vi "RPC Method PerformOCVMeasurement.vi"(8 "error in (no error)":errorcluster, 11 "OOP Server in":refnum<class "OCV2.lvclass">) -> (0 "error out":errorcluster, 3 "OOP Server out":refnum<class "OCV2.lvclass">)   [LabVIEW 2019, in "OCV2.lvlib" / "OCV2.lvclass"]
uses:
  OCV2.lvclass
  OCV2.lvclass/OCV2.ctl
  RPC Messages/measurementservice_ErrorOut/measurementservice_ErrorOut_Data.ctl
  RPC Messages/measurementservice_OCVRaw/measurementservice_OCVRaw_Data.ctl
  RPC Messages/measurementservice_OCVData/measurementservice_OCVData_Data.ctl
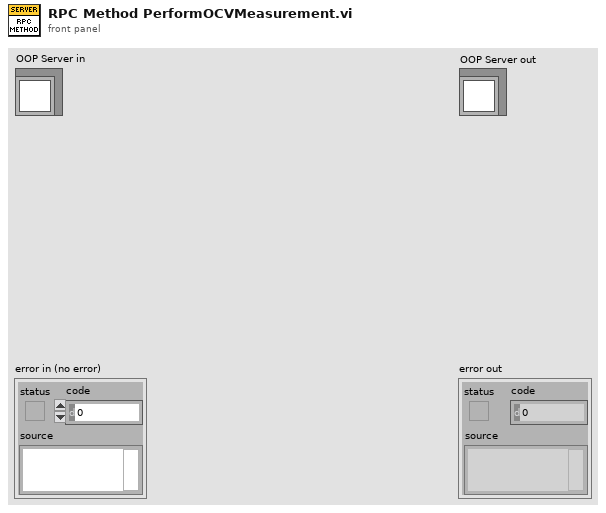
[diagram p1: front panel]
types:
  T1 = typedef "OCV2.lvlib/OCV2.lvclass/measurementservice_OCVData_Data.ctl" = cluster{"data":T2[]}
  T2 = typedef "OCV2.lvlib/OCV2.lvclass/measurementservice_OCVRaw_Data.ctl" = cluster{"battery1voltage":sgl, "battery2voltage":sgl, "battery3voltage":sgl, "battery4voltage":sgl, "battery5voltage":sgl, "battery6voltage":sgl, "battery7voltage":sgl, "battery8voltage":sgl, "battery9voltage":sgl, "battery10voltage":sgl, "battery11voltage":sgl, "battery12voltage":sgl, "battery13voltage":sgl, "battery14voltage":sgl, "battery15voltage":sgl, "battery16voltage":sgl, "battery17voltage":sgl, "battery18voltage":sgl, "battery19voltage":sgl, "battery20voltage":sgl, "battery21voltage":sgl, "battery22voltage":sgl, "battery23voltage":sgl, "battery24voltage":sgl, "error":T3}
  T3 = typedef "OCV2.lvlib/OCV2.lvclass/measurementservice_ErrorOut_Data.ctl" = cluster{"errCode":i32, "errMessage":string}
  T4 = typedef "OCV2.lvlib/OCV2.lvclass/Server Internal UEs.ctl" = cluster{"Invoke Internal UE":refnum<user-event>, "Query Internal UE":refnum<user-event>, "PerformOCVMeasurement Internal UE":refnum<user-event>, "PerformACIRMeasurement Internal UE":refnum<user-event>, "StreamOCVMeasurement Internal UE":refnum<user-event>, "Register Internal UE":refnum<user-event>}
  T5 = typedef "OCV2.lvlib/OCV2.lvclass/Server gRPC UEs.ctl" = cluster{"Invoke gRPC UE":refnum<user-event>, "Query gRPC UE":refnum<user-event>, "PerformOCVMeasurement gRPC UE":refnum<user-event>, "PerformACIRMeasurement gRPC UE":refnum<user-event>, "StreamOCVMeasurement gRPC UE":refnum<user-event>, "Register gRPC UE":refnum<user-event>}
  T6 = typedef "OCV2.lvlib/gprc-lvsupport.lvlib/grpcId.ctl" = u64
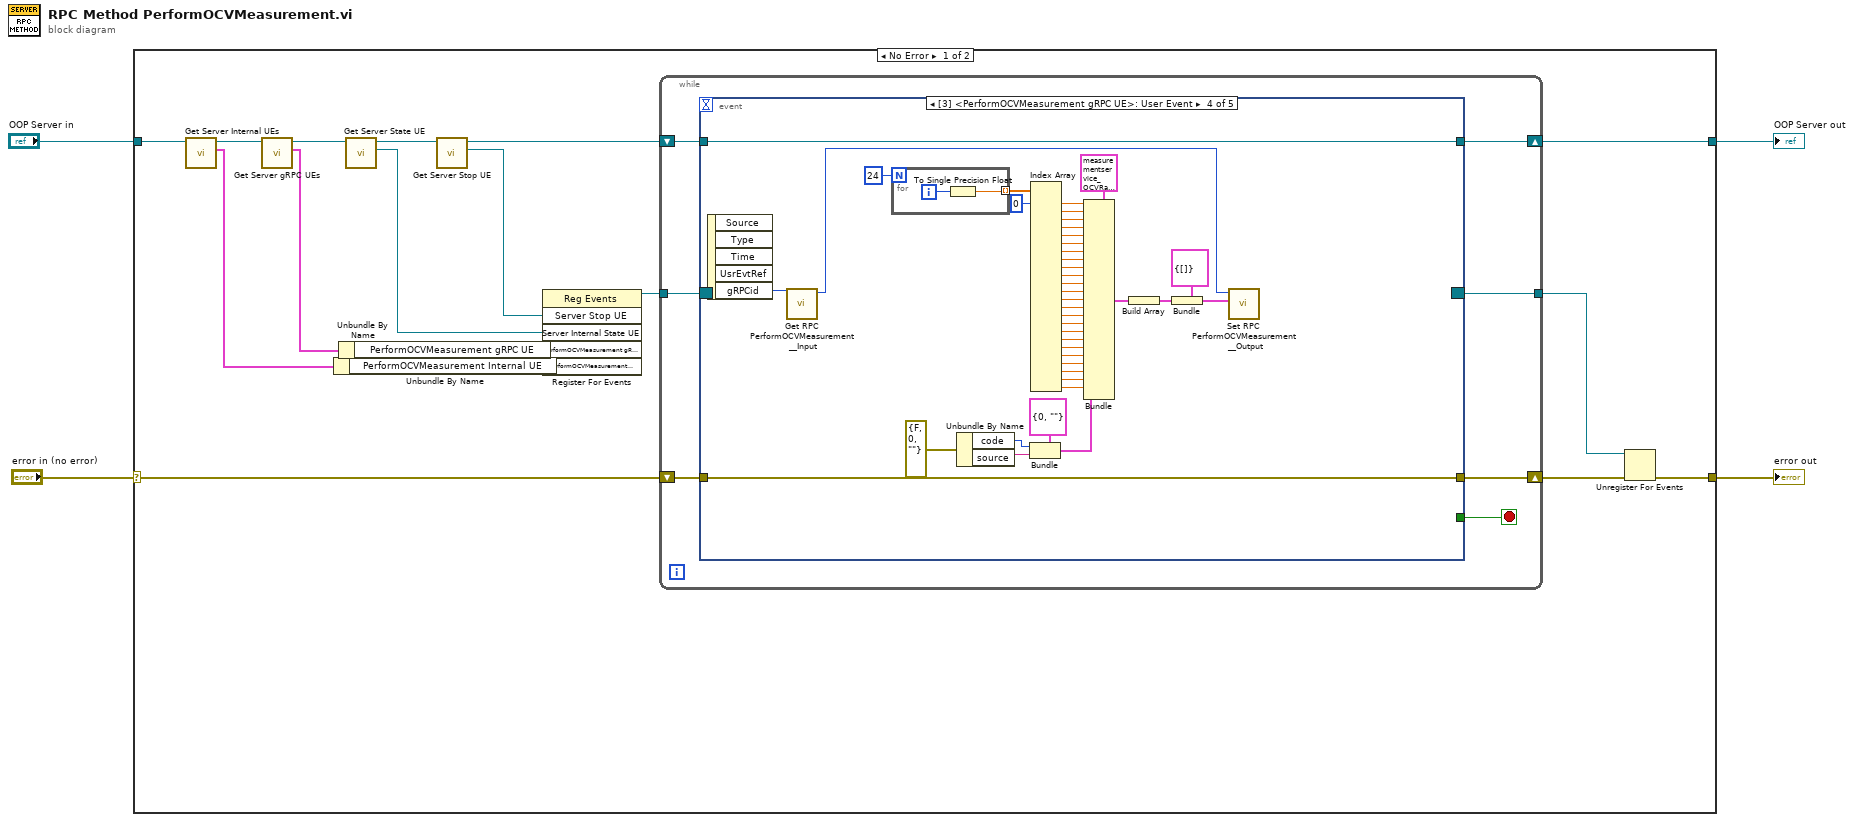
[diagram p0: block diagram]
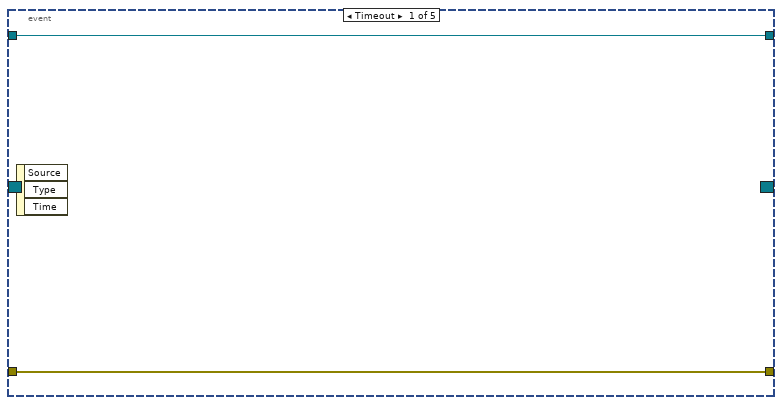
[diagram p2: hidden frame]
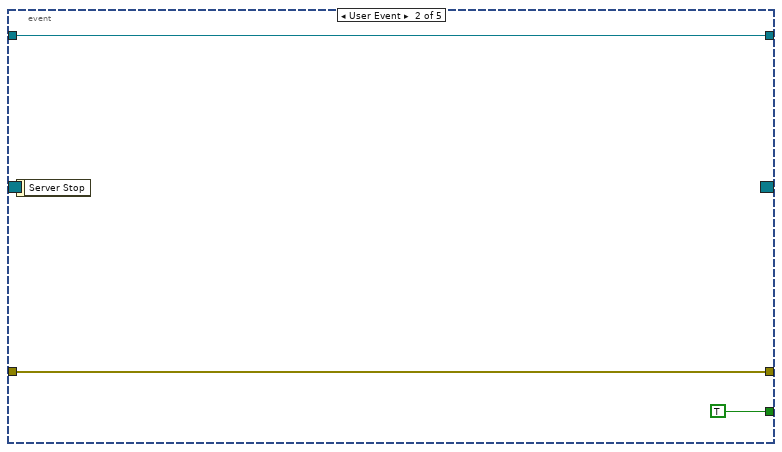
[diagram p3: hidden frame]
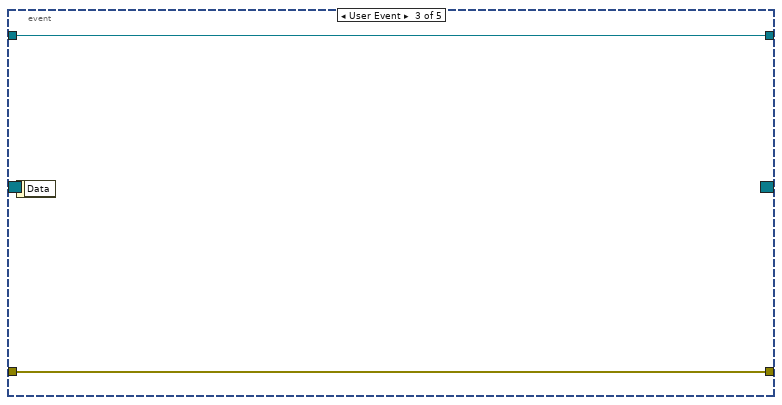
[diagram p4: hidden frame]
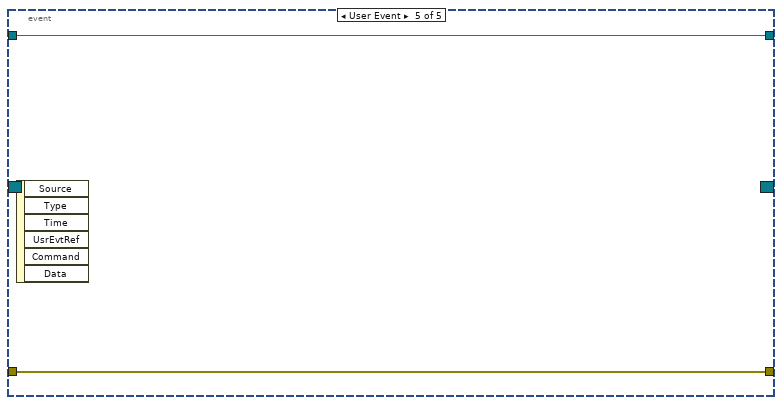
[diagram p5: hidden frame]
diagram:
  n1 = case shown="No Error" "error in (no error)" {
    selector: "error in (no error)" -> [w17 w82]
    tunnel: [w15 w82] -> w3
    tunnel: "OOP Server in" -> [w19 w81]
    tunnel: [w5 w81] -> w1
    frame No Error {
      n2 = call "Get Server Internal UEs.vi"("OOP Server in"=w19) -> ("Server Internal UEs"=w11:T4, "OOP Server out"=w18:refnum<class "OCV2.lvclass">)  [unwired: 9 in]
      n3 = call "Get Server gRPC UEs.vi"("OOP Server in"=w18) -> ("Server gRPC UEs"=w13:T5, "OOP Server out"=w8:refnum<class "OCV2.lvclass">)  [unwired: 9 in]
      n4 = Unbundle By Name ("Unbundle Internal UE")(w11) -> ("PerformOCVMeasurement Internal UE"=w10:refnum<user-event>)
      n5 = Unbundle By Name ("Unbundle gRPC UE")(w13) -> ("PerformOCVMeasurement gRPC UE"=w12:refnum<user-event>)
      n6 = call "Get Server State UE.vi"("Template Server in"=w8) -> ("Server Internal State UE"=w6:refnum<user-event>, "Template Server out"=w7:refnum<class "OCV2.lvclass">)  [unwired: 9 in]
      n7 = call "Get Server Stop UE.vi"("OOP Server in"=w7) -> ("Server Stop UE"=w21:refnum<user-event>, "OOP Server out"=w9:refnum<class "OCV2.lvclass">)  [unwired: 9 in]
      n8 = register-events(w21, w6, w12, w10) -> (reference out=w20:refnum<event-registration>)  [unwired: 2 in, 1 out]
      n9 = while {
        tunnel: w20 -> [w28]
        tunnel: [w24] -> w14
        shift-right: [w25] -> w16
        shift-left: w17 -> [w26]
        shift-right: [w22] -> w5
        shift-left: w9 -> [w23]
        stop <- w27 stop-if-true
        n10 = event "RPC Method Event Structure" shown="[3] <PerformOCVMeasurement gRPC UE>: User Event" {
          selector: w28 -> [_ _ _ _ _]
          dyn-events: [_ _ _ _ _] -> w24
          timeout: _ -> [_ _ _ _ _]
          tunnel: [_ TRUE _ _ _] -> w27
          tunnel: w26 -> [w30 w32 w35 w76 w80]
          tunnel: [w30 w32 w35 w76 w80] -> w25
          tunnel: w23 -> [w29 w31 w34 w75 w79]
          tunnel: [w29 w31 w34 w75 w79] -> w22
          event Timeout {
            n11 = event-data() -> ()  [unwired: 1 in, 3 out]
          }
          event User Event {
            n12 = event-data() -> ()  [unwired: 1 in, 1 out]
          }
          event User Event {
            n13 = event-data() -> ()  [unwired: 1 in, 1 out]
          }
          event User Event {
            n14 = event-data() -> ("gRPCid"=w42:T6)  [unwired: 1 in, 4 out]
            n15 = call "Get RPC PerformOCVMeasurement __Input.vi"("gRPCid in"=w42) -> ("gRPCid out"=w41:T6)  [unwired: 8 in, 2 out]
            n16 = for {
              N: 24 -> [_]
              tunnel: [w78] -> w45 mode=indexing
              i -> [w77]
              n17 = To Single Precision Float(number=w77) -> (single precision float=w78:sgl)
            }
            n18 = Unbundle By Name(errorcluster {"status"=FALSE, "code"=0, "source"=""} ("input cluster")) -> ("code"=w72:i32, "source"=w71:string)
            n19 = Bundle(cluster=T3 {"errCode"=0, "errMessage"=""} ("measurementservice_ErrorOut_Data"), "errCode"=w72, "errMessage"=w71) -> (w70:T3)
            n20 = Index Array(array=w45, index #1=0 ("index")) -> (element #1=w69:sgl, element #2=w68:sgl, element #3=w67:sgl, element #4=w66:sgl, element #5=w65:sgl, element #6=w64:sgl, element #7=w63:sgl, element #8=w62:sgl, element #9=w61:sgl, element #10=w60:sgl, element #11=w59:sgl, element #12=w58:sgl, element #13=w57:sgl, element #14=w56:sgl, element #15=w55:sgl, element #16=w54:sgl, element #17=w53:sgl, element #18=w52:sgl, element #19=w51:sgl, element #20=w50:sgl, element #21=w49:sgl, element #22=w48:sgl, element #23=w47:sgl, element #24=w46:sgl)  [unwired: 23 in]
            n21 = Bundle(cluster=T2 {"battery1voltage"=0.0, "battery2voltage"=0.0, "battery3voltage"=0.0, "battery4voltage"=0.0, "battery5voltage"=0.0, "battery6voltage"=0.0, "battery7voltage"=0.0, "battery8voltage"=0.0, "battery9voltage"=0.0, "battery10voltage"=0.0, "battery11voltage"=0.0, "battery12voltage"=0.0, "battery13voltage"=0.0, "battery14voltage"=0.0, "battery15voltage"=0.0, "battery16voltage"=0.0, "battery17voltage"=0.0, "battery18voltage"=0.0, "battery19voltage"=0.0, "battery20voltage"=0.0, "battery21voltage"=0.0, "battery22voltage"=0.0, "battery23voltage"=0.0, "battery24voltage"=0.0, "error"={"errCode"=0, "errMessage"=""}} ("measurementservice_OCVRaw_Data"), "battery1voltage"=w69, "battery2voltage"=w68, "battery3voltage"=w67, "battery4voltage"=w66, "battery5voltage"=w65, "battery6voltage"=w64, "battery7voltage"=w63, "battery8voltage"=w62, "battery9voltage"=w61, "battery10voltage"=w60, "battery11voltage"=w59, "battery12voltage"=w58, "battery13voltage"=w57, "battery14voltage"=w56, "battery15voltage"=w55, "battery16voltage"=w54, "battery17voltage"=w53, "battery18voltage"=w52, "battery19voltage"=w51, "battery20voltage"=w50, "battery21voltage"=w49, "battery22voltage"=w48, "battery23voltage"=w47, "battery24voltage"=w46, "error"=w70) -> (w73:T2)
            n22 = Build Array(w73) -> (w74:T2[])
            n23 = Bundle(cluster=T1 {"data"=[]} ("measurementservice_OCVData_Data"), "data"=w74) -> (w36:T1)
            n24 = call "Set RPC PerformOCVMeasurement __Output.vi"("Message Data"=w36, "gRPCid in"=w41) -> ()  [unwired: 9 in, 1 out]
          }
          event User Event {
            n25 = event-data() -> ()  [unwired: 1 in, 6 out]
          }
        }
      }
      n26 = Unregister For Events(event registration refnum=w14, error in=w16) -> (error out=w15:errorcluster)
    }
    frame Error {
    }
  }
  "error out" <- w3
  "OOP Server out" <- w1
